vi "VisaRead.vi"(8 "error out":errorcluster, 11 "VISA resource name in":refnum<visa-resource-name>) -> (0 "error out":errorcluster, 2 "output":string, 3 "VISA resource name out":refnum<visa-resource-name>)   [LabVIEW 2020]
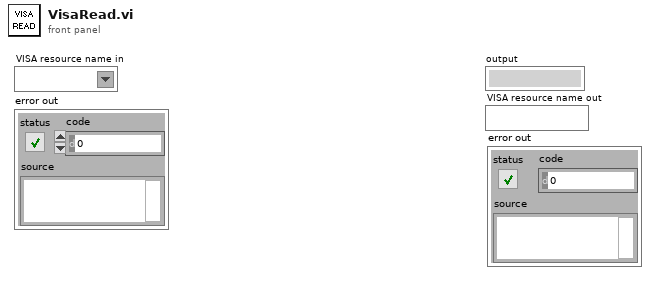
[diagram p1: front panel]
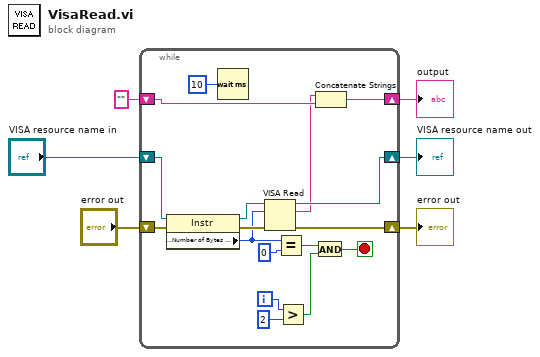
[diagram p0: block diagram]
diagram:
  n1 = while {
    shift-right: [w22] -> w5
    shift-left: "VISA resource name in" -> [w21]
    shift-right: [w23] -> w6
    shift-left: "error out" -> [w18]
    shift-right: [w17] -> w4
    shift-left: "" -> [w16]
    i -> [w8]
    stop <- w11 stop-if-true
    n2 = property class="Instr"(reference=w21, error in=w18) -> (reference out=w20:refnum<visa-resource-name>, error out=w19:errorcluster, "Serial Settings:Number of Bytes at Serial Port"=w14:u32)
    n3 = Wait (ms)(milliseconds to wait=u32 10) -> ()  [unwired: 1 out]
    n4 = VISA Read(VISA resource name=w20, byte count=w14, error in (no error)=w19) -> (VISA resource name out=w22:refnum<visa-resource-name>, read buffer=w15:string, error out=w23:errorcluster)  [unwired: 1 out]
    n5 = Equal?(x=w14, y=u32 0) -> (x = y?=w10:bool)
    n6 = Greater?(x=w8, y=2 ("x")) -> (0:w9:bool)
    n7 = And(x=w10, y=w9) -> (x .and. y?=w11:bool)
    n8 = Concatenate Strings(w15, w16) -> (w17:string)
  }
  "output" <- w4
  "VISA resource name out" <- w5
  "error out" <- w6
